vi "Parse Category from Frame Name.vi"(11 "Frame Name":string) -> (2 "is a Category?":bool, 3 "Category Name":string)   [LabVIEW 2013, in "JKI State Machine API.lvlib" / "JKI SM.lvclass"]
uses:
  JKI SM.lvclass
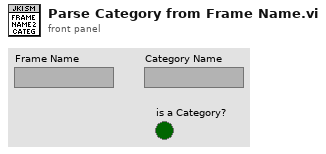
[diagram p1: front panel]
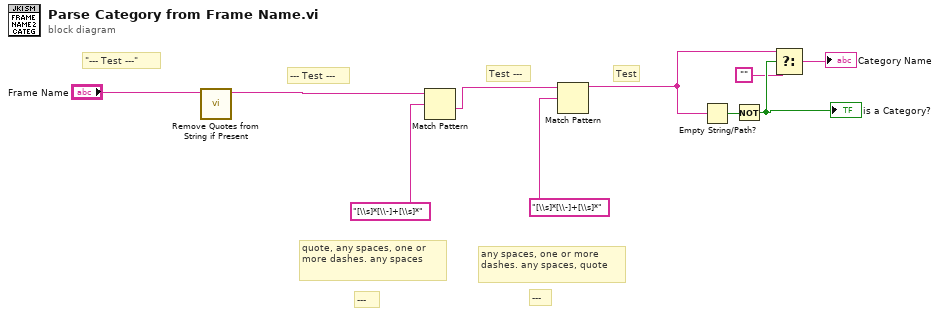
[diagram p0: block diagram]
diagram:
  # "--- Test ---"
  # "---"
  # "---"
  # "Test"
  # "Test ---"
  # "\"--- Test ---\""
  # "any spaces, one or more dashes. any spaces, quote"
  # "quote, any spaces, one or more dashes. any spaces"
  n1 = call "Remove Quotes from String if Present.vi"("String"="Frame Name") -> ("String with Quotes Removed"=w1:string)  [unwired: 10 in]
  n2 = Match Pattern(string=w1, regular expression="[\\s]*[\\-]+[\\s]*") -> (after substring=w8:string)  [unwired: 1 in, 3 out]
  n3 = Match Pattern(string=w8, regular expression="[\\s]*[\\-]+[\\s]*") -> (before substring=w7:string)  [unwired: 1 in, 3 out]
  n4 = Empty String/Path?(string/path=w7) -> (empty?=w10:bool)
  n5 = Not(x=w10) -> (.not. x?=w5:bool)
  "is a Category?" <- w5
  n6 = Select(t=w7, s=w5, f="") -> (s? t:f=→"Category Name":string)
